vi "Rio_Move_XY (DONE).vi"(8 "Error In":errorcluster, 9 "Home Position":dbl[](array[numeric]), 10 "Coordinate":dbl[](array[numeric]), 11 "Home/Coordinate (T/F)":bool) -> (0 "Error Out":errorcluster, 4 "Output Charts":T1, 5 "Stop":bool)   [LabVIEW 2017]
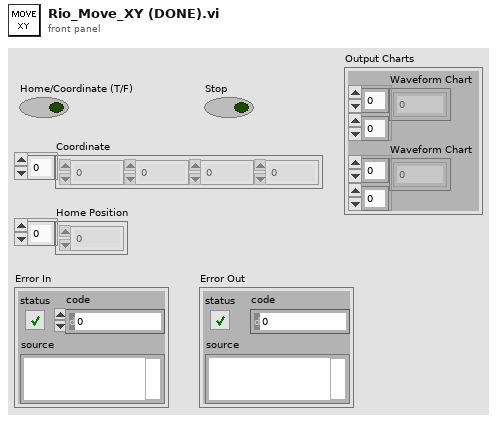
[diagram p1: front panel]
types:
  T1 = cluster{"Waveform Chart":dbl[][], "Waveform Chart":dbl[][]}
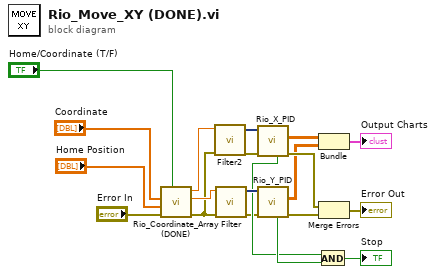
[diagram p0: block diagram]
diagram:
  n1 = call "Rio_Coordinate_Array (DONE).vi"("Coordinate Selection"="Home/Coordinate (T/F)", "Error In"="Error In", "Home Position"="Home Position", "Coordinate"="Coordinate") -> ("Error Out"=w2:errorcluster, "Y"=w18:dbl, "X"=w1:dbl)  [unwired: 5 in]
  n2 = call "Filter2"("error in (no error)"=w2, "Signal"=w1) -> ("error out"=w3:errorcluster, "Filtered Signal"=w4:dynamicdata)  [unwired: 8 in]
  n3 = call "Filter"("error in (no error)"=w2, "Signal"=w18) -> ("error out"=w8:errorcluster, "Filtered Signal"=w13:dynamicdata)  [unwired: 8 in]
  n4 = call "Rio_X_PID.vi"("Error In"=w3, "Setpoint"=w4) -> ("Error Out"=w9:errorcluster, "Waveform Chart"=w7:dbl[][], "Stop"=w11:bool)  [unwired: 6 in, 1 out]
  n5 = call "Rio_Y_PID.vi"("Error In"=w8, "Setpoint"=w13) -> ("Error Out"=w10:errorcluster, "Waveform Chart"=w6:dbl[][], "Stop"=w12:bool)  [unwired: 6 in, 1 out]
  n6 = And(x=w11, y=w12) -> (x .and. y?=→"Stop":bool)
  n7 = Bundle("Waveform Chart"=w7, "Waveform Chart"=w6) -> (→"Output Charts":T1)  [unwired: 1 in]
  n8 = Merge Errors(w9, w10) -> (→"Error Out":errorcluster)
